vi "test ChemTrac.vi"() -> ()   [LabVIEW 2019]
panel:
  in  "HF1 2":dbl[](array[numeric])=[1.0]
  out "NTU1 2":dbl
  in  "Boolean 2":bool
  in  "Boolean":bool
  out "NTU1":dbl
  in  "HF1":dbl[](array[numeric])=[1.0]
  out "output value 2":dbl
  in  "Set Points 2":dbl[](array[numeric])=[0.0]
  out "elapsed time (s)":dbl format="%_19f"
  out "Set Point names":string[](array[string])=["data interval (s)", "com port number", "device ID", "data address"]
  out "output value":dbl
  out "x/y":dbl
  out "Numeric":i32
  in  "stop":bool
  in  "Set Points":dbl[](array[numeric])=[5.0, 5.0, 1.0]
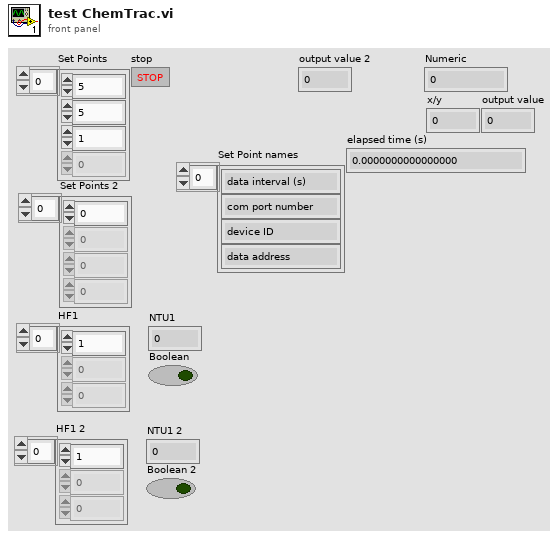
[diagram p1: front panel]
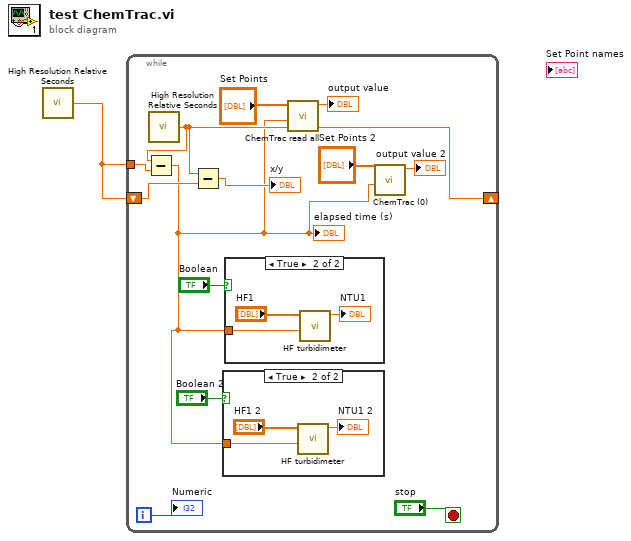
[diagram p0: block diagram]
diagram:
  n1 = call <vilib>:"High Resolution Relative Seconds.vi"() -> ("relative seconds"=w1:dbl)
  n2 = while {
    shift-right: [w8] -> _
    shift-left: w1 -> [w9]
    tunnel: w1 -> [w7]
    i -> [w12]
    stop <- "stop" stop-if-true
    n3 = call <vilib>:"High Resolution Relative Seconds.vi"() -> ("relative seconds"=w8:dbl)
    n4 = Subtract(x=w8, y=w7) -> (x-y=w2:dbl)
    "elapsed time (s)" <- w2
    n5 = Subtract(x=w8, y=w9) -> (x-y=→"x/y":dbl)
    n6 = case shown="True" "Boolean 2" {
      tunnel: w2 -> [_ w16]
      frame False {
      }
      frame True {
        n7 = call "HF turbidimeter.vi"("Time"=w16, "Set Points"="HF1 2") -> ("output value"=→"NTU1 2":dbl)  [unwired: 4 in, 1 out]
      }
    }
    n8 = case shown="True" "Boolean" {
      tunnel: w2 -> [_ w19]
      frame False {
      }
      frame True {
        n9 = call "HF turbidimeter.vi"("Time"=w19, "Set Points"="HF1") -> ("output value"=→"NTU1":dbl)  [unwired: 4 in, 1 out]
      }
    }
    n10 = call "ChemTrac read all.vi"("Time"=w2, "Set Points"="Set Points") -> ("output value"=→"output value":dbl)  [unwired: 4 in, 1 out]
    n11 = call "ChemTrac (0).vi"("Time"=w2, "Set Points"="Set Points 2") -> ("output value"=→"output value 2":dbl)  [unwired: 4 in, 1 out]
    "Numeric" <- w12
  }
